vi "Read ADC_UI Actor.vi"(8 "error in (no error)":errorcluster, 11 "UI Actor in":refnum<class "UI Actor.lvclass">) -> (0 "error out":errorcluster, 3 "UI Actor out":refnum<class "UI Actor.lvclass">)   [LabVIEW 2020, in "UI Actor.lvlib" / "UI Actor.lvclass"]
uses:
  UI Actor.lvclass
  UI Actor.lvclass/UI Actor.ctl
  Abstract/Serial Device/Serial Device.lvclass
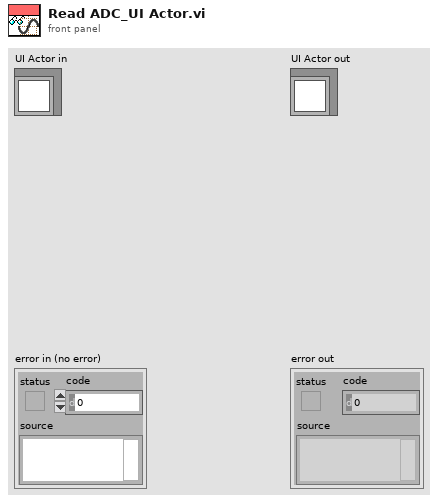
[diagram p1: front panel]
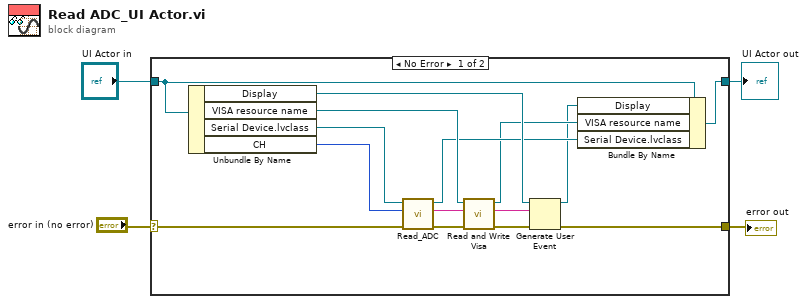
[diagram p0: block diagram]
diagram:
  n1 = case shown="No Error" "error in (no error)" {
    selector: "error in (no error)" -> [w8 w20]
    tunnel: [w6 w21] -> w2
    tunnel: "UI Actor in" -> [w9 w21]
    tunnel: [w7 w20] -> w1
    frame No Error {
      n2 = Unbundle By Name(w9) -> ("Display"=w13:refnum<user-event>, "VISA resource name"=w14:refnum<visa-resource-name>, "Serial Device.lvclass"=w15:refnum<class "Serial Device.lvclass">, "CH"=w5:i32)
      n3 = call-dynamic "Read_ADC.vi"("error in (no error)"=w8, "CH"=w5, "Serial Device in"=w15) -> ("error out"=w17:errorcluster, "Command to Send"=w19:string, "Serial Device out"=w12:refnum<class "Serial Device.lvclass">)  [unwired: 5 in, 1 out]
      n4 = call "Read and Write Visa.vi"("error in (no error)"=w17, "Command to Send"=w19, "VISA Refnum in"=w14) -> ("error out"=w16:errorcluster, "Expected Response out"=w18:string, "VISA Refnum out"=w11:refnum<visa-resource-name>)  [unwired: 6 in]
      n5 = Generate User Event(user event=w13, event data cluster=w18, error in=w16) -> (user event out=w10:refnum<user-event>, error out=w7:errorcluster)  [unwired: 1 in]
      n6 = Bundle By Name(cluster=w9, "Display"=w10, "VISA resource name"=w11, "Serial Device.lvclass"=w12) -> (w6:refnum<class "UI Actor.lvclass">)
    }
    frame Error {
    }
  }
  "error out" <- w1
  "UI Actor out" <- w2
